vi "Pre-Build VI - Run Unit Tests.vi"(8 "error in (no error)":errorcluster) -> (0 "error out":errorcluster, 1 "VIs without test coverage":string[](array[string]), 2 "error type":enum16{"fatal", "non-fatal", "warning"}(ring), 3 "Failed Tests":string[](array[string]))   [LabVIEW 2009]
uses:
  <userlib>/_OpenG.lib/array/array.llb/Conditional Auto-Indexing Tunnel (String)__ogtk.vi
  <userlib>/_OpenG.lib/array/array.llb/Filter 1D Array (String)__ogtk.vi
panel:
  in  "type specifier VI Refnum (for type only)":refnum<vi>
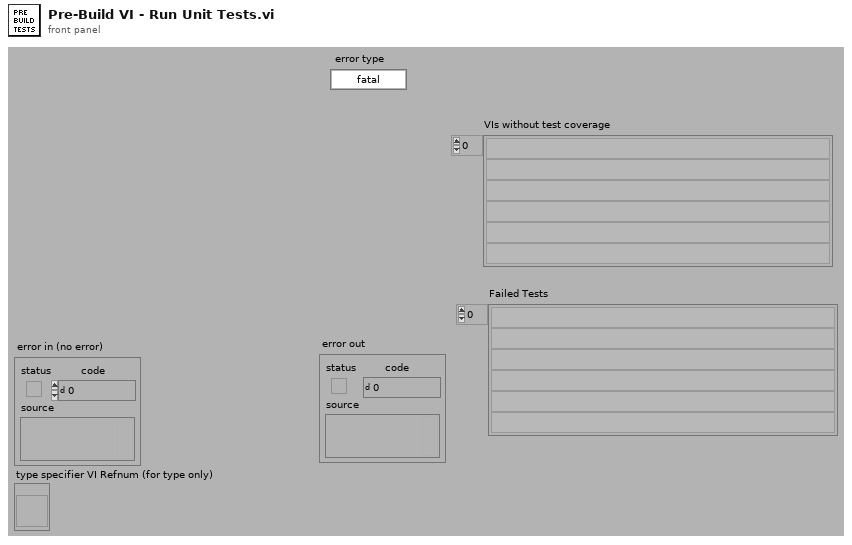
[diagram p1: front panel]
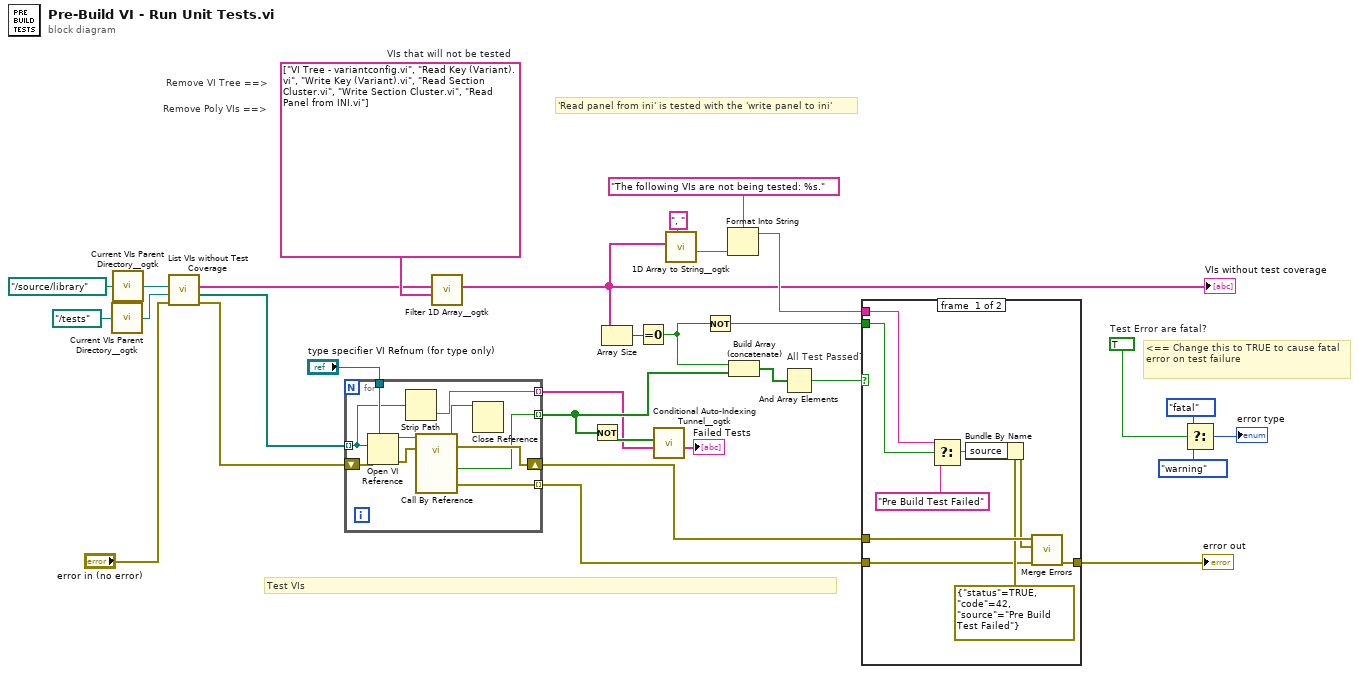
[diagram p0: block diagram]
diagram:
  w18 = TRUE  # Test Error are fatal?
  w29 = string[] ["VI Tree - variantconfig.vi", "Read Key (Variant).vi", "Write Key (Variant).vi", "Read Section Cluster.vi", "Write Section Cluster.vi", "Read Panel from INI.vi"]  # VIs that will not be tested
  # "'Read panel from ini' is tested with the 'write panel to ini'"
  # "<== Change this to TRUE to cause fatal error on test failure"
  # "Remove Poly VIs ==>"
  # "Remove VI Tree ==>"
  # "All Test Passed?"
  # "Test VIs"
  n1 = call <userlib>:"Current VIs Parent Directory__ogtk.vi"("Relative path (.)"=path "../tests") -> ("Parent Directory (+ Relative)"=w13:path)  [unwired: 4 in]
  n2 = call <userlib>:"Current VIs Parent Directory__ogtk.vi"("Relative path (.)"=path "../source/library") -> ("Parent Directory (+ Relative)"=w22:path)  [unwired: 4 in]
  n3 = call "List VIs without Test Coverage.vi"("error in (no error)"="error in (no error)", "Tests Root"=w13, "Source Root"=w22) -> ("error out"=w9:errorcluster, "Test VIs"=w12:path[], "VIs without test coverage"=w28:string[])  [unwired: 6 in]
  n4 = for {
    tunnel: w12 -> [w33] mode=indexing
    tunnel: "type specifier VI Refnum (for type only)" -> [w41]
    shift-right: [w38] -> w10
    shift-left: w9 -> [w37]
    tunnel: [w36] -> w4 mode=indexing
    tunnel: [w34] -> w8 mode=indexing
    tunnel: [w32] -> w2 mode=indexing
    n5 = Open VI Reference(type specifier VI Refnum (for type only)=w41, vi path=w33, error in (no error)=w37) -> (vi reference=w40:refnum<vi>, error out=w39:errorcluster)  [unwired: 3 in]
    n6 = Strip Path(path=w33) -> (name=w32:string)  [unwired: 1 out]
    n7 = call-by-ref "?"(reference=w40, error in=w39) -> (reference out=w35:refnum<vi>, error out=w38:errorcluster, 0:"error out"=w34:errorcluster, "pass"=w36:bool)  [unwired: 10 in]
    n8 = Close Reference(reference=w35) -> ()  [unwired: 1 in, 1 out]
  }
  n9 = call-poly <userlib>:"Filter 1D Array__ogtk.vi"("items to filter"=w29, "array"=w28) -> ("filtered array"=w7:string[])  [unwired: 4 in, 1 out]
  "VIs without test coverage" <- w7
  n10 = Not(x=w4) -> (.not. x?=w3:bool[])
  n11 = Array Size(array=w7) -> (size(s)=w6:i32)
  n12 = Equal To 0?(x=w6) -> (x = 0?=w5:bool)
  n13 = call-poly <userlib>:"Conditional Auto-Indexing Tunnel__ogtk.vi"("Array in"=w2, "Elements to keep"=w3) -> ("Filtered Array out"=→"Failed Tests":string[])  [unwired: 5 in]
  n14 = call <userlib>:"1D Array to String__ogtk.vi"("delimiter (Tab)"=", ", "Array of Strings"=w7) -> ("delimited string"=w26:string)  [unwired: 9 in]
  n15 = Not(x=w5) -> (.not. x?=w23:bool)
  n16 = Format Into String(format string="The following VIs are not being tested: %s.", w26) -> (resulting string=w24:string)  [unwired: 2 in, 1 out]
  n17 = Build Array (concatenate)(w5, w4) -> (w31:bool[])
  n18 = And Array Elements(Boolean array=w31) -> (logical AND=w30:bool)
  n19 = case shown="False" w30 {
    tunnel: w10 -> [w50 w51]
    tunnel: [w49 w51] -> w20
    tunnel: w23 -> [w48 _]
    tunnel: w24 -> [w47 _]
    tunnel: w8 -> [w42 _]
    frame #0 {
      n20 = Select(t=w47, s=w48, f="Pre Build Test Failed" ("source")) -> (s? t:f=w45:string)
      n21 = Bundle By Name(cluster=errorcluster {"status"=TRUE, "code"=42, "source"="Pre Build Test Failed"} ("error out"), "source"=w45) -> (w44:errorcluster)
      n22 = call <vilib>:"Merge Errors.vi"("error array in"=w42, "error in 2 (no error)"=w44, "error in 1 (no error)"=w50) -> ("error out"=w49:errorcluster)  [unwired: 4 in]
    }
    frame #1 {
    }
  }
  "error out" <- w20
  n23 = Select(t=enum16{"fatal", "non-fatal", "warning"}."fatal" ("error type"), s=w18, f=enum16{"fatal", "non-fatal", "warning"}."warning" ("error type")) -> (s? t:f=→"error type":enum16{"fatal", "non-fatal", "warning"})
